vi "Determine More Warnings.vi"(6 "Max Wind Speed":dbl, 7 "Current Wind Speed":dbl, 8 "error in (no error)":errorcluster, 9 "Min Temp":dbl, 10 "Max Temp":dbl, 11 "Current Temp":dbl) -> (0 "error out":errorcluster, 1 "Warning?":bool, 2 "Warning Text":string)   [LabVIEW 2014]
uses:
  Det Warnings.ctl
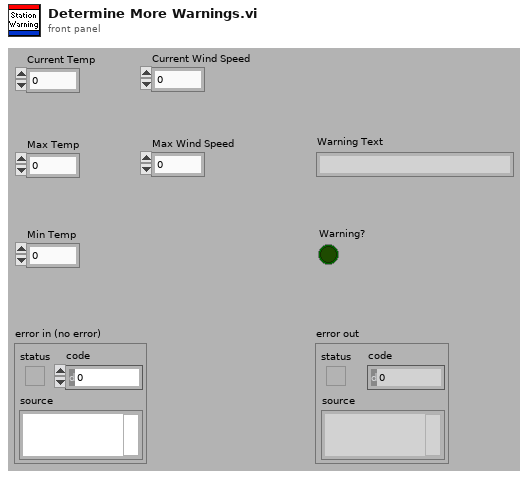
[diagram p1: front panel]
types:
  T1 = typedef "Det Warnings.ctl" = enum16{"Heatstroke", "Freeze", "High Wind", "Generate Warning", "Error Check"}
  T2 = cluster{"Current Temp":dbl, "Max Temp":dbl, "Min Temp":dbl, "Current Wind Speed":dbl, "Max Wind Speed":dbl}
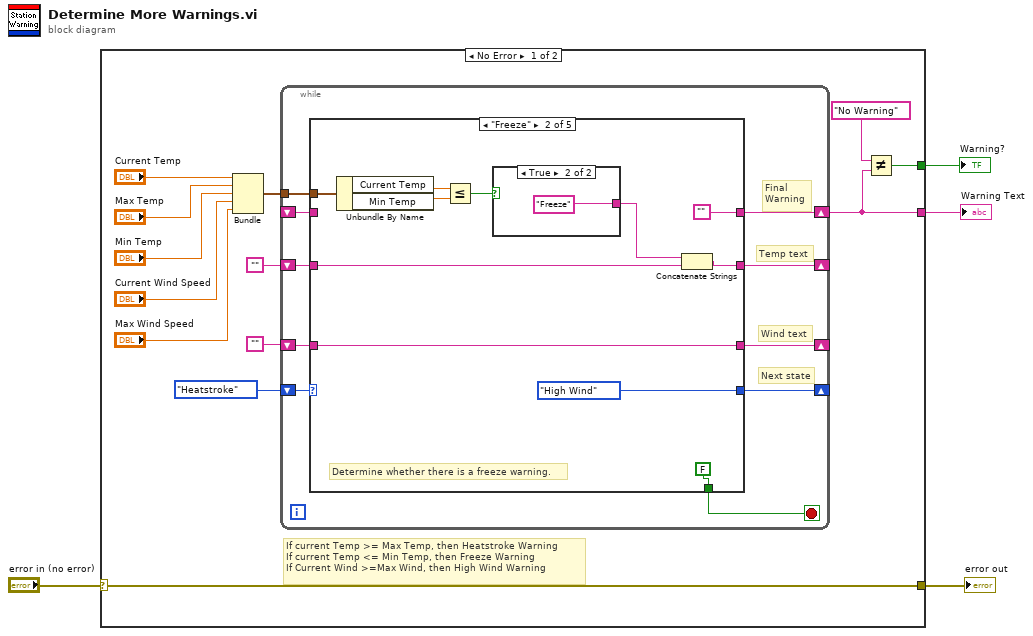
[diagram p0: block diagram]
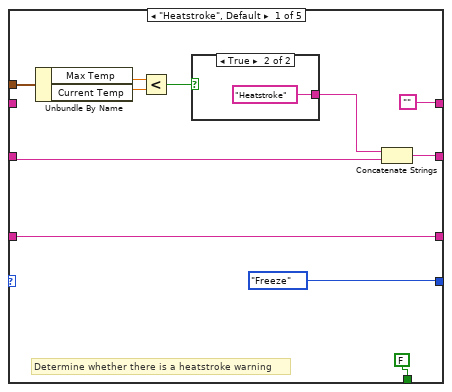
[diagram p2: hidden frame]
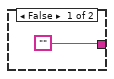
[diagram p3: hidden frame]
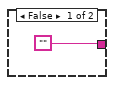
[diagram p4: hidden frame]
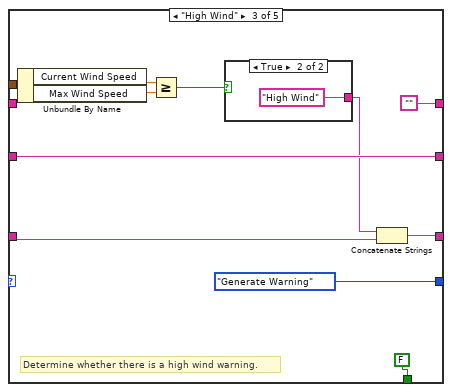
[diagram p5: hidden frame]
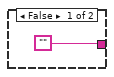
[diagram p6: hidden frame]
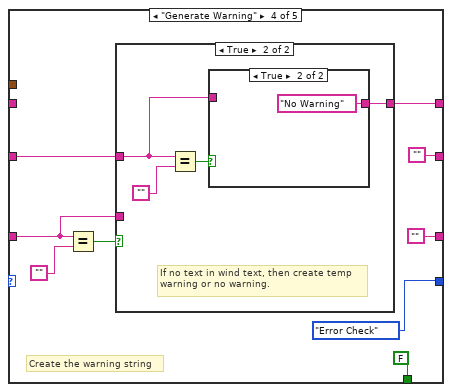
[diagram p7: hidden frame]
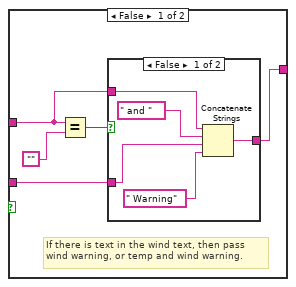
[diagram p8: hidden frame]
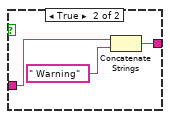
[diagram p9: hidden frame]
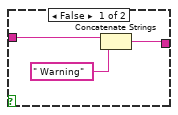
[diagram p10: hidden frame]
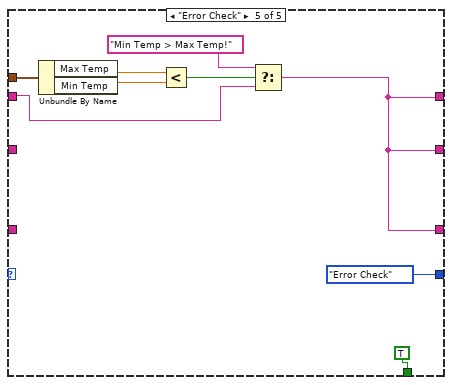
[diagram p11: hidden frame]
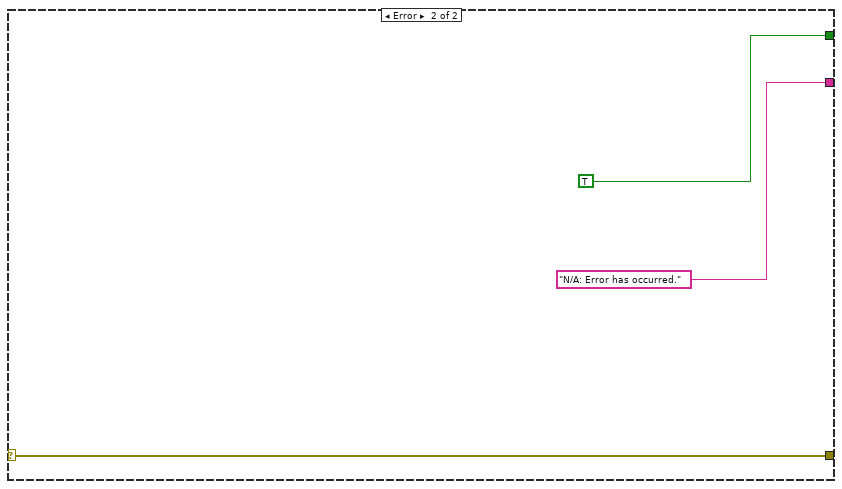
[diagram p12: hidden frame]
diagram:
  n1 = case shown="No Error" "error in (no error)" {
    selector: "error in (no error)" -> [w16 w108]
    tunnel: [w16 w108] -> w3
    tunnel: [w17 TRUE] -> w2
    tunnel: [w6 "N/A: Error has occurred." ("f")] -> w1
    frame No Error {
      # "If current Temp >= Max Temp, then Heatstroke Warning\nIf current Temp <= Min Temp, then Freeze Warning\nIf Current Wind >=Max Wind, then High Wind Warning"
      n2 = Bundle("Current Temp"="Current Temp", "Max Temp"="Max Temp", "Min Temp"="Min Temp", "Current Wind Speed"="Current Wind Speed", "Max Wind Speed"="Max Wind Speed") -> (w9:T2)  [unwired: 1 in]
      n3 = while {
        tunnel: w9 -> [w24]
        shift-right: [w23] -> _
        shift-left: Det_Warnings."Heatstroke" ("Enum") -> [w27]
        shift-right: [w26] -> _
        shift-left: "" -> [w22]
        shift-right: [w25] -> _
        shift-left: "" -> [w21]
        shift-right: [w20] -> w6
        shift-left: _ -> [w18]
        stop <- w19 stop-if-true
        # "Final\nWarning"
        # "Next state"
        # "Wind text"
        # "Temp text"
        n4 = case shown="\"Freeze\"" w27 {
          tunnel: [w30 w46 w58 "" w99] -> w25
          tunnel: [w33 w45 w59 "" w99] -> w26
          tunnel: w24 -> [w37 w51 w64 _ w105]
          tunnel: [Det_Warnings."Freeze" ("Enum") Det_Warnings."High Wind" ("Enum") Det_Warnings."Generate Warning" ("Enum") Det_Warnings."Error Check" ("Enum") Det_Warnings."Error Check" ("Enum")] -> w23
          tunnel: w22 -> [w32 w43 w59 w75 _]
          tunnel: w21 -> [w30 w46 w56 w72 _]
          tunnel: ["" "" "" w71 w99] -> w20
          tunnel: [FALSE FALSE FALSE FALSE TRUE] -> w19
          tunnel: w18 -> [_ _ _ _ w101]
          frame "Heatstroke", Default {
            # "Determine whether there is a heatstroke warning"
            n5 = Unbundle By Name(w37) -> ("Max Temp"=w36:dbl, "Current Temp"=w35:dbl)
            n6 = Less?(x=w36, y=w35) -> (x < y?=w38:bool)
            n7 = case shown="True" w38 {
              tunnel: ["" "Heatstroke"] -> w31
              frame False {
              }
              frame True {
              }
            }
            n8 = Concatenate Strings(w31, w32) -> (w33:string)
          }
          frame "Freeze" {
            # "Determine whether there is a freeze warning."
            n9 = Unbundle By Name(w51) -> ("Current Temp"=w49:dbl, "Min Temp"=w48:dbl)
            n10 = Less Or Equal?(x=w49, y=w48) -> (x <= y?=w50:bool)
            n11 = case shown="True" w50 {
              tunnel: ["" "Freeze"] -> w44
              frame False {
              }
              frame True {
              }
            }
            n12 = Concatenate Strings(w44, w43) -> (w45:string)
          }
          frame "High Wind" {
            # "Determine whether there is a high wind warning."
            n13 = Unbundle By Name(w64) -> ("Current Wind Speed"=w63:dbl, "Max Wind Speed"=w62:dbl)
            n14 = Greater Or Equal?(x=w63, y=w62) -> (x >= y?=w61:bool)
            n15 = case shown="True" w61 {
              tunnel: ["" "High Wind"] -> w57
              frame False {
              }
              frame True {
              }
            }
            n16 = Concatenate Strings(w57, w56) -> (w58:string)
          }
          frame "Generate Warning" {
            # "Create the warning string"
            n17 = Equal?(x=w72, y="") -> (x = y?=w73:bool)
            n18 = case shown="True" w73 {
              tunnel: [w78 w92] -> w71
              tunnel: w75 -> [w76 w89]
              tunnel: w72 -> [w77 _]
              frame False {
                # "If there is text in the wind text, then pass\nwind warning, or temp and wind warning."
                n19 = Equal?(x=w76, y="") -> (x = y?=w79:bool)
                n20 = case shown="False" w79 {
                  tunnel: [w83 w87] -> w78
                  tunnel: w77 -> [w82 w86]
                  tunnel: w76 -> [w81 _]
                  frame False {
                    n21 = Concatenate Strings(w81, " and " ("string"), w82, " Warning" ("string")) -> (w83:string)
                  }
                  frame True {
                    n22 = Concatenate Strings(w86, " Warning" ("string")) -> (w87:string)
                  }
                }
              }
              frame True {
                # "If no text in wind text, then create temp\nwarning or no warning."
                n23 = Equal?(x=w89, y="") -> (x = y?=w90:bool)
                n24 = case shown="True" w90 {
                  tunnel: [w95 "No Warning"] -> w92
                  tunnel: w89 -> [w94 _]
                  frame False {
                    n25 = Concatenate Strings(w94, " Warning") -> (w95:string)
                  }
                  frame True {
                  }
                }
              }
            }
          }
          frame "Error Check" {
            n26 = Unbundle By Name(w105) -> ("Max Temp"=w104:dbl, "Min Temp"=w103:dbl)
            n27 = Less?(x=w104, y=w103) -> (x < y?=w102:bool)
            n28 = Select(t="Min Temp > Max Temp!", s=w102, f=w101) -> (s? t:f=w99:string)
          }
        }
      }
      n29 = Not Equal?(x="No Warning", y=w6) -> (x != y?=w17:bool)
    }
    frame Error {
    }
  }
  "error out" <- w3
  "Warning Text" <- w1
  "Warning?" <- w2
